vi "Prepare Rope Grid.vi"(0 "Offset":cdb, 1 "Columns":i32, 2 "Positions":T1, 5 "Rows":i32) -> (6 "Rope":cluster{dbl, dbl}[](array[cluster]), 7 "Rope Grid":cluster{"Grid":string, "H Direction":string})   [LabVIEW 2020, in "AoC 2022.lvlib"]
uses:
  AoC 2022.lvlib
  Positions.ctl
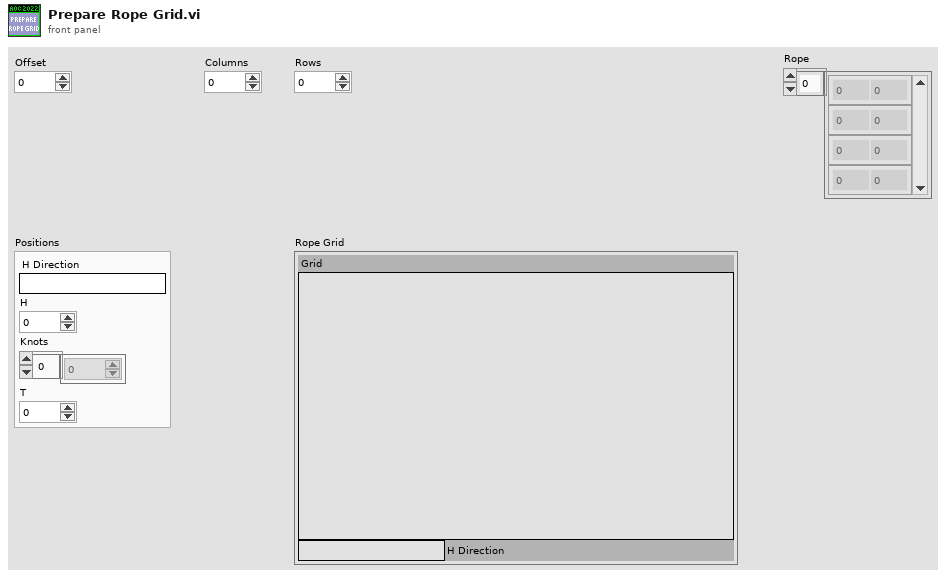
[diagram p1: front panel]
types:
  T1 = typedef "AoC 2022.lvlib/Positions.ctl" = cluster{"H Direction":string, "H":cdb, "Knots":cdb[], "T":cdb}
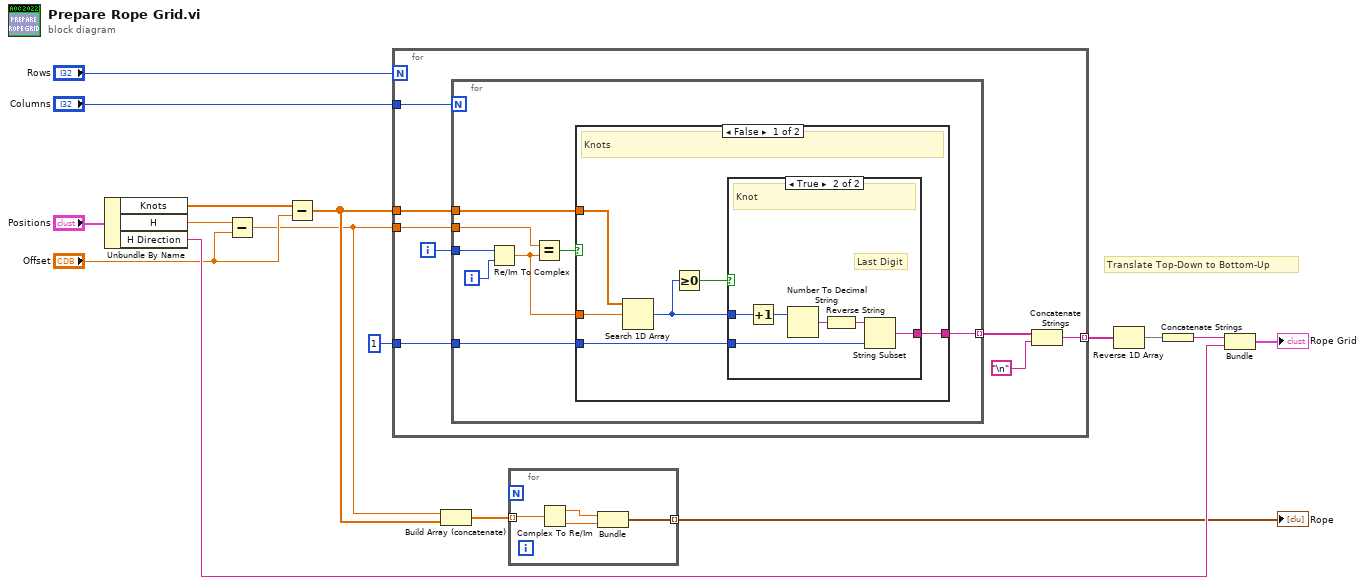
[diagram p0: block diagram]
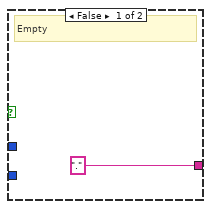
[diagram p2: hidden frame]
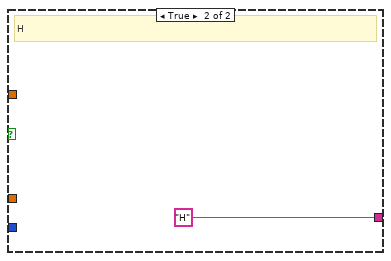
[diagram p3: hidden frame]
diagram:
  # "Translate Top-Down to Bottom-Up"
  n1 = Unbundle By Name("Positions") -> ("Knots"=w10:cdb[], "H"=w13:cdb, "H Direction"=w15:string)
  n2 = Subtract(x=w13, y="Offset") -> (x-y=w4:cdb)
  n3 = Subtract(x=w10, y="Offset") -> (x-y=w5:cdb[])
  n4 = for {
    N: "Rows" -> [_]
    tunnel: "Columns" -> [w24]
    tunnel: w4 -> [w23]
    tunnel: w5 -> [w21]
    tunnel: [w19] -> w12 mode=indexing
    tunnel: 1 -> [w17]
    i -> [w22]
    n5 = for {
      N: w24 -> [_]
      tunnel: w23 -> [w30]
      tunnel: w22 -> [w31]
      tunnel: w21 -> [w28]
      tunnel: [w26] -> w20 mode=indexing
      tunnel: w17 -> [w25]
      i -> [w32]
      n6 = Re/Im To Complex(1:w32, 2:w31) -> (0:w29:cdb)
      n7 = Equal?(x=w30, y=w29) -> (x = y?=w27:bool)
      n8 = case shown="False" w27 {
        tunnel: w29 -> [w38 _]
        tunnel: w28 -> [w37 _]
        tunnel: [w36 "H"] -> w26
        tunnel: w25 -> [w33 _]
        frame False {
          # "Knots"
          n9 = Search 1D Array(1D array=w37, element=w38) -> (index of element=w35:i32)  [unwired: 1 in]
          n10 = Greater Or Equal To 0?(x=w35) -> (x >= 0?=w34:bool)
          n11 = case shown="True" w34 {
            tunnel: w35 -> [_ w44]
            tunnel: ["." w42] -> w36
            tunnel: w33 -> [_ w40]
            frame False {
              # "Empty"
            }
            frame True {
              # "Last Digit"
              # "Knot"
              n12 = Increment(x=w44) -> (x+1=w45:i32)
              n13 = Number To Decimal String(number=w45) -> (decimal integer string=w43:string)  [unwired: 1 in]
              n14 = Reverse String(1:w43) -> (0:w41:string)
              n15 = String Subset(string=w41, length (rest)=w40) -> (substring=w42:string)  [unwired: 1 in]
            }
          }
        }
        frame True {
          # "H"
        }
      }
    }
    n16 = Concatenate Strings(w20, "\n") -> (w19:string)
  }
  n17 = Build Array (concatenate)(w4, w5) -> (w3:cdb[])
  n18 = for {
    tunnel: w3 -> [w50] mode=indexing
    tunnel: [w47] -> w2 mode=indexing
    n19 = Complex To Re/Im(x + iy=w50) -> (x=w49:dbl, y=w48:dbl)
    n20 = Bundle(w49, w48) -> (w47:cluster{dbl, dbl})  [unwired: 1 in]
  }
  "Rope" <- w2
  n21 = Reverse 1D Array(array=w12) -> (reversed array=w14:string[])
  n22 = Concatenate Strings(w14) -> (w11:string)
  n23 = Bundle(w11, "H Direction"=w15) -> (→"Rope Grid":cluster{string, "H Direction":string})  [unwired: 1 in]
